vi "档位加载比例 (子VI).vi"(10 "更换车型加载比例":dbl, 11 "D1-D3/R1/R2加载比例":dbl) -> (3 "数值":dbl)   [LabVIEW 2016]
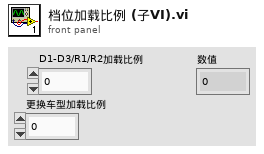
[diagram p1: front panel]
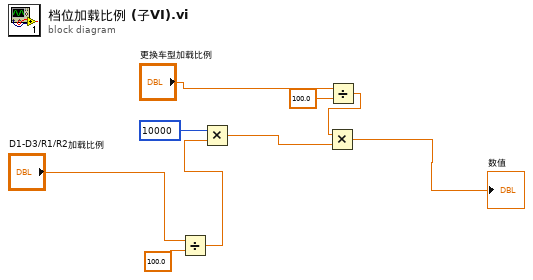
[diagram p0: block diagram]
diagram:
  n1 = Divide(x="D1-D3/R1/R2加载比例", y=100.0) -> (x/y=w9:dbl)
  n2 = Multiply(x=i16 10000 ("D1扭矩给定"), y=w9) -> (x*y=w1:dbl)
  n3 = Divide(x="更换车型加载比例", y=100.0) -> (x/y=w2:dbl)
  n4 = Multiply(x=w2, y=w1) -> (x*y=→"数值":dbl)
